vi "Parse CIF File from ATK.vi"(11 "CIF File from ATK":path) -> (3 "Atomic Structure":T1={"Structure Name"="ATK-generated POSCAR  \r\n", "Lattice vector a"=[6.48, 0.0, 0.0], "Lattice vector b"=[0.0, 6.48, 0.0], "Lattice vector c"=[0.0, 0.0, 32.4], "Atoms Array"=[{"Atom Name"="", "Positions (Direct)"=[[0.0, 0.0, 0.0005805493563561], [0.5, 0.5, 0.0005805493563561], [0.5, 0.0, 0.1012044869316679], [0.0, 0.5, 0.1012044869316679], [0.0, 0.0, 0.201657427297086], [0.5, 0.5, 0.201657427297086], [0.5, 0.0, 0.3022756106216986], [0.0, 0.5, 0.3022756106216986], [0.25, 0.25, 0.3937799251008503], [0.75, 0.75, 0.3937799251008503], [0.75, 0.25, 0.5004577122084005], [0.25, 0.75, 0.5004577122084005], [0.0, 0.0, 0.5916454825280393], [0.5, 0.5, 0.5916454825280393], [0.5, 0.0, 0.6986135219684406], [0.0, 0.5, 0.6986135219684406], [0.0, 0.0, 0.7992442554474246], [0.5, 0.5, 0.7992442554474246], [0.5, 0.0, 0.8999316304227629], [0.0, 0.5, 0.8999316304227629]], "Positions (Cartesian)"=[[0.0, 0.0, 0.0005805493563561], [0.5, 0.5, 0.0005805493563561], [0.5, 0.0, 0.1012044869316679], [0.0, 0.5, 0.1012044869316679], [0.0, 0.0, 0.201657427297086], [0.5, 0.5, 0.201657427297086], [0.5, 0.0, 0.3022756106216986], [0.0, 0.5, 0.3022756106216986], [0.25, 0.25, 0.3937799251008503], [0.75, 0.75, 0.3937799251008503], [0.75, 0.25, 0.5004577122084005], [0.25, 0.75, 0.5004577122084005], [0.0, 0.0, 0.5916454825280393], [0.5, 0.5, 0.5916454825280393], [0.5, 0.0, 0.6986135219684406], [0.0, 0.5, 0.6986135219684406], [0.0, 0.0, 0.7992442554474246], [0.5, 0.5, 0.7992442554474246], [0.5, 0.0, 0.8999316304227629], [0.0, 0.5, 0.8999316304227629]]}, {"Atom Name"="", "Positions (Direct)"=[[0.25, 0.25, 0.0508700657751452], [0.75, 0.75, 0.0508700657751452], [0.75, 0.25, 0.1514314226755048], [0.25, 0.75, 0.1514314226755048], [0.25, 0.25, 0.2516943562152962], [0.75, 0.75, 0.2516943562152962], [0.75, 0.25, 0.356312302565805], [0.25, 0.75, 0.356312302565805], [0.0, 0.0, 0.4497768887256497], [0.5, 0.5, 0.4497768887256497], [0.5, 0.0, 0.553935227460559], [0.0, 0.5, 0.553935227460559], [0.25, 0.25, 0.6478094902292927], [0.75, 0.75, 0.6478094902292927], [0.75, 0.25, 0.7489441399571884], [0.25, 0.75, 0.7489441399571884], [0.25, 0.25, 0.8495690683463202], [0.75, 0.75, 0.8495690683463202], [0.75, 0.25, 0.9502664361665122], [0.25, 0.75, 0.9502664361665122]], "Positions (Cartesian)"=[[0.25, 0.25, 0.0508700657751452], [0.75, 0.75, 0.0508700657751452], [0.75, 0.25, 0.1514314226755048], [0.25, 0.75, 0.1514314226755048], [0.25, 0.25, 0.2516943562152962], [0.75, 0.75, 0.2516943562152962], [0.75, 0.25, 0.356312302565805], [0.25, 0.75, 0.356312302565805], [0.0, 0.0, 0.4497768887256497], [0.5, 0.5, 0.4497768887256497], [0.5, 0.0, 0.553935227460559], [0.0, 0.5, 0.553935227460559], [0.25, 0.25, 0.6478094902292927], [0.75, 0.75, 0.6478094902292927], [0.75, 0.25, 0.7489441399571884], [0.25, 0.75, 0.7489441399571884], [0.25, 0.25, 0.8495690683463202], [0.75, 0.75, 0.8495690683463202], [0.75, 0.25, 0.9502664361665122], [0.25, 0.75, 0.9502664361665122]]}], "# of atoms"=40})   [LabVIEW 2010]
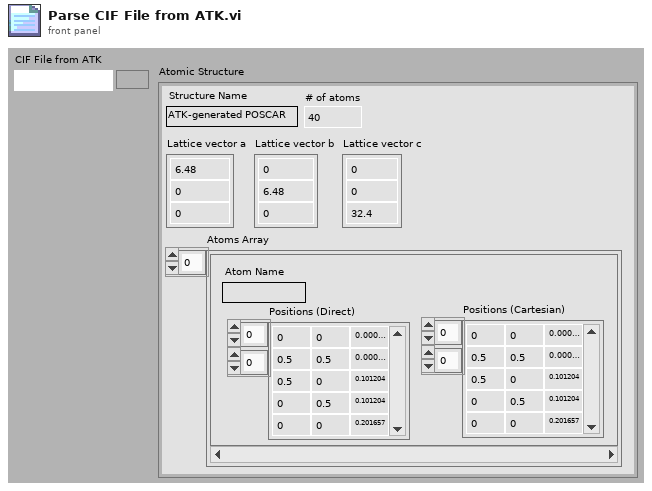
[diagram p1: front panel]
types:
  T1 = cluster{"Structure Name":string, "Lattice vector a":dbl[], "Lattice vector b":dbl[], "Lattice vector c":dbl[], "Atoms Array":cluster{"Atom Name":string, "Positions (Direct)":dbl[][], "Positions (Cartesian)":dbl[][]}[], "# of atoms":i32}
  T2 = cluster{"Atom Name":string, "Positions (Direct)":dbl[][], "Positions (Cartesian)":dbl[][]}[]
  T3 = cluster{"token string":string, "Positions (Direct)":dbl[][], "Positions (Cartesian)":dbl[][]}[]
  T4 = cluster{"Atom Name":string, "Positions (Direct)":dbl[][], "Positions (Cartesian)":dbl[][]}
  T5 = cluster{"name":string, dbl[], dbl[], dbl[], "Atoms Array":cluster{"Atom Name":string, "Positions (Direct)":dbl[][], "Positions (Cartesian)":dbl[][]}[], i32}
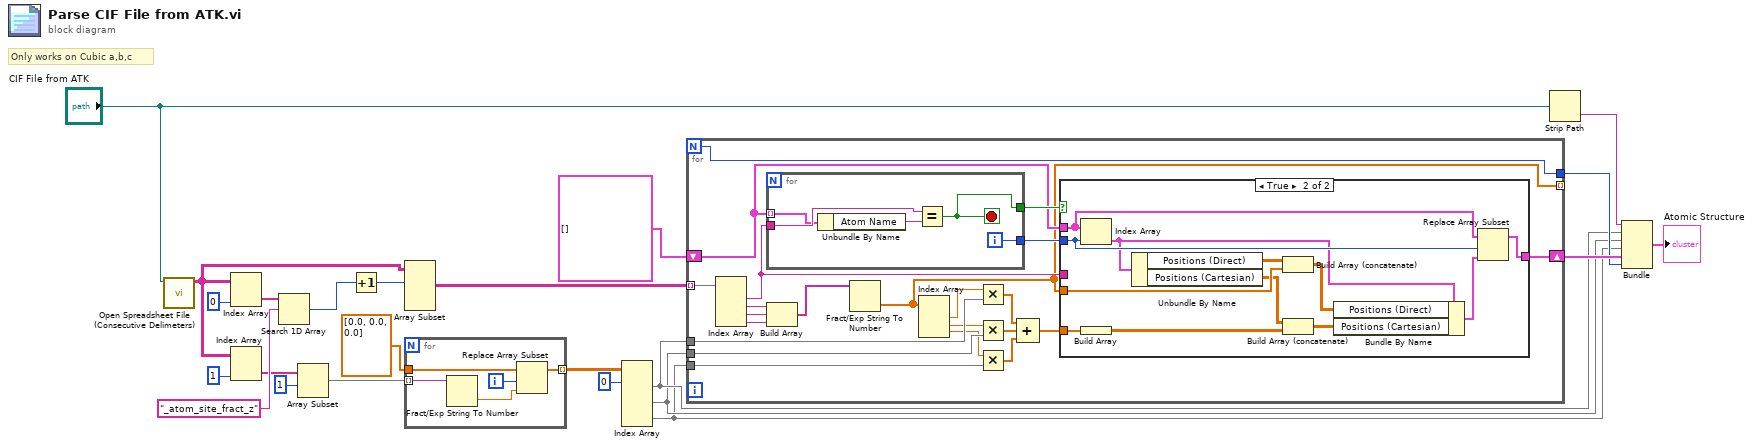
[diagram p0: block diagram]
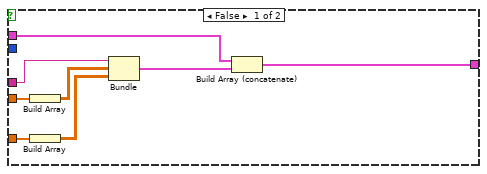
[diagram p2: hidden frame]
diagram:
  # "Only works on Cubic a,b,c"
  n1 = call "Open Spreadsheet File (Consecutive Delimeters).vi"("File"="CIF File from ATK") -> ("Array"=w15:string[][])  [unwired: 9 in, 1 out]
  n2 = Index Array(array=w15, index (col)=0 ("disabled index (col)")) -> (element=w22:string[])  [unwired: 1 in]
  n3 = Index Array(array=w15, index (col)=1 ("disabled index (col)")) -> (element=w14:string[])  [unwired: 1 in]
  n4 = Search 1D Array(1D array=w22, element="_atom_site_fract_z") -> (index of element=w20:i32)  [unwired: 1 in]
  n5 = Array Subset(array=w14, index=1) -> (w12:string[])  [unwired: 1 in]
  n6 = Increment(x=w20) -> (x+1=w19:i32)
  n7 = Array Subset(array=w15, index (row)=w19) -> (w18:string[][])  [unwired: 3 in]
  n8 = for {
    tunnel: w12 -> [w28] mode=indexing
    tunnel: [w25] -> w10 mode=indexing
    tunnel: dbl[] [0.0, 0.0, 0.0] -> [w24]
    i -> [w27]
    n9 = Fract/Exp String To Number(string=w28) -> (number=w26:dbl)  [unwired: 3 in, 1 out]
    n10 = Replace Array Subset(array=w24, new element=w26, index=w27) -> (w25:dbl[])
  }
  n11 = Index Array(array=w10, index (row) #1=0 ("index (row)")) -> (element #1=w3:dbl[], element #2=w2:dbl[], element #3=w1:dbl[])  [unwired: 5 in]
  n12 = for {
    N -> [w45]
    tunnel: w18 -> [w50] mode=indexing
    shift-right: [w41] -> w8
    shift-left: T2 [] ("Atoms Array") -> [w42]
    tunnel: [w36] -> _ mode=indexing
    tunnel: [w45] -> w4
    tunnel: w3 -> [w39]
    tunnel: w2 -> [w38]
    tunnel: w1 -> [w37]
    n13 = Index Array(array=w50) -> (element #1=w43:string, element #2=w49:string, element #3=w48:string, element #4=w47:string)  [unwired: 4 in]
    n14 = for {
      tunnel: w42 -> [w74] mode=indexing
      tunnel: w43 -> [w75]
      tunnel: [w72] -> w40
      tunnel: [w71] -> w44
      i -> [w72]
      stop <- w71 stop-if-true
      n15 = Unbundle By Name(w74) -> ("Atom Name"=w73:string)
      n16 = Equal?(x=w75, y=w73) -> (x = y?=w71:bool)
    }
    n17 = Build Array(w49, w48, w47) -> (w46:string[])
    n18 = Fract/Exp String To Number(string=w46) -> (number=w36:dbl[])  [unwired: 3 in, 1 out]
    n19 = Index Array(array=w36) -> (element #1=w35:dbl, element #2=w34:dbl, element #3=w33:dbl)  [unwired: 3 in]
    n20 = Multiply(x=w35, y=w39) -> (x*y=w32:dbl[])
    n21 = Multiply(x=w34, y=w38) -> (x*y=w31:dbl[])
    n22 = Multiply(x=w33, y=w37) -> (x*y=w30:dbl[])
    n23 = Compound Arithmetic op=ADD(w32, w31, w30) -> (w29:dbl[])
    n24 = case shown="True" w44 {
      tunnel: w36 -> [w58 w66]
      tunnel: w43 -> [w57 _]
      tunnel: w42 -> [w56 w70]
      tunnel: [w53 w63] -> w41
      tunnel: w40 -> [_ w69]
      tunnel: w29 -> [w52 w62]
      frame False {
        n25 = Build Array(w58) -> (w55:dbl[][])
        n26 = Build Array(w52) -> (w51:dbl[][])
        n27 = Bundle("token string"=w57, w55, w51) -> (w54:cluster{"token string":string, dbl[][], dbl[][]})  [unwired: 1 in]
        n28 = Build Array (concatenate)(w56, w54) -> (w53:T3)
      }
      frame True {
        n29 = Index Array(array=w70, index=w69) -> (element=w68:T4)
        n30 = Build Array(w62) -> (w60:dbl[][])
        n31 = Unbundle By Name(w68) -> ("Positions (Direct)"=w67:dbl[][], "Positions (Cartesian)"=w61:dbl[][])
        n32 = Build Array (concatenate)(w67, w66) -> (w65:dbl[][])
        n33 = Build Array (concatenate)(w61, w60) -> (w59:dbl[][])
        n34 = Bundle By Name(cluster=w68, "Positions (Direct)"=w65, "Positions (Cartesian)"=w59) -> (w64:T4)
        n35 = Replace Array Subset(array=w70, new element=w64, index=w69) -> (w63:T2)
      }
    }
  }
  n36 = Strip Path(path="CIF File from ATK") -> (name=w6:string)  [unwired: 1 out]
  n37 = Bundle("name"=w6, w3, w2, w1, "Atoms Array"=w8, w4) -> (→"Atomic Structure":T5)  [unwired: 1 in]
